vi "Initialise.vi"(8 "error in (no error)":errorcluster, 11 "Actor in":refnum<class "Main View.lvclass">) -> (0 "error out":errorcluster, 3 "Actor out":refnum<class "Main View.lvclass">, 5 "Observers":T1)   [LabVIEW 2015, in "Main View.lvclass"]
uses:
  Main View.lvclass
  Re-use Libraries/Minimal Actor Framework/Messaging/Message/Message.lvclass
  Re-use Libraries/Minimal Actor Framework/Actors/Base Actor/Actor/Update User Event.ctl
  Re-use Libraries/Utility/Utility.lvlib
  Actors/Main Controller/Actor/Main Controller Actor.lvclass
  Re-use Libraries/Minimal Actor Framework/Actors/Base Actor/Actor/Actor.lvclass
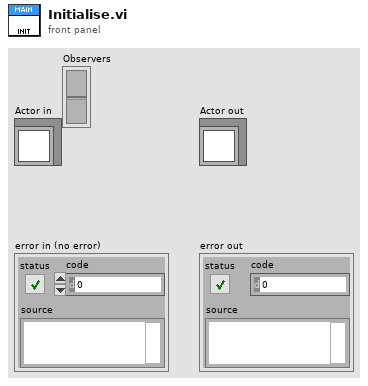
[diagram p1: front panel]
types:
  T1 = cluster{"Actor":refnum<event-registration>, "Main Controller":refnum<event-registration>}
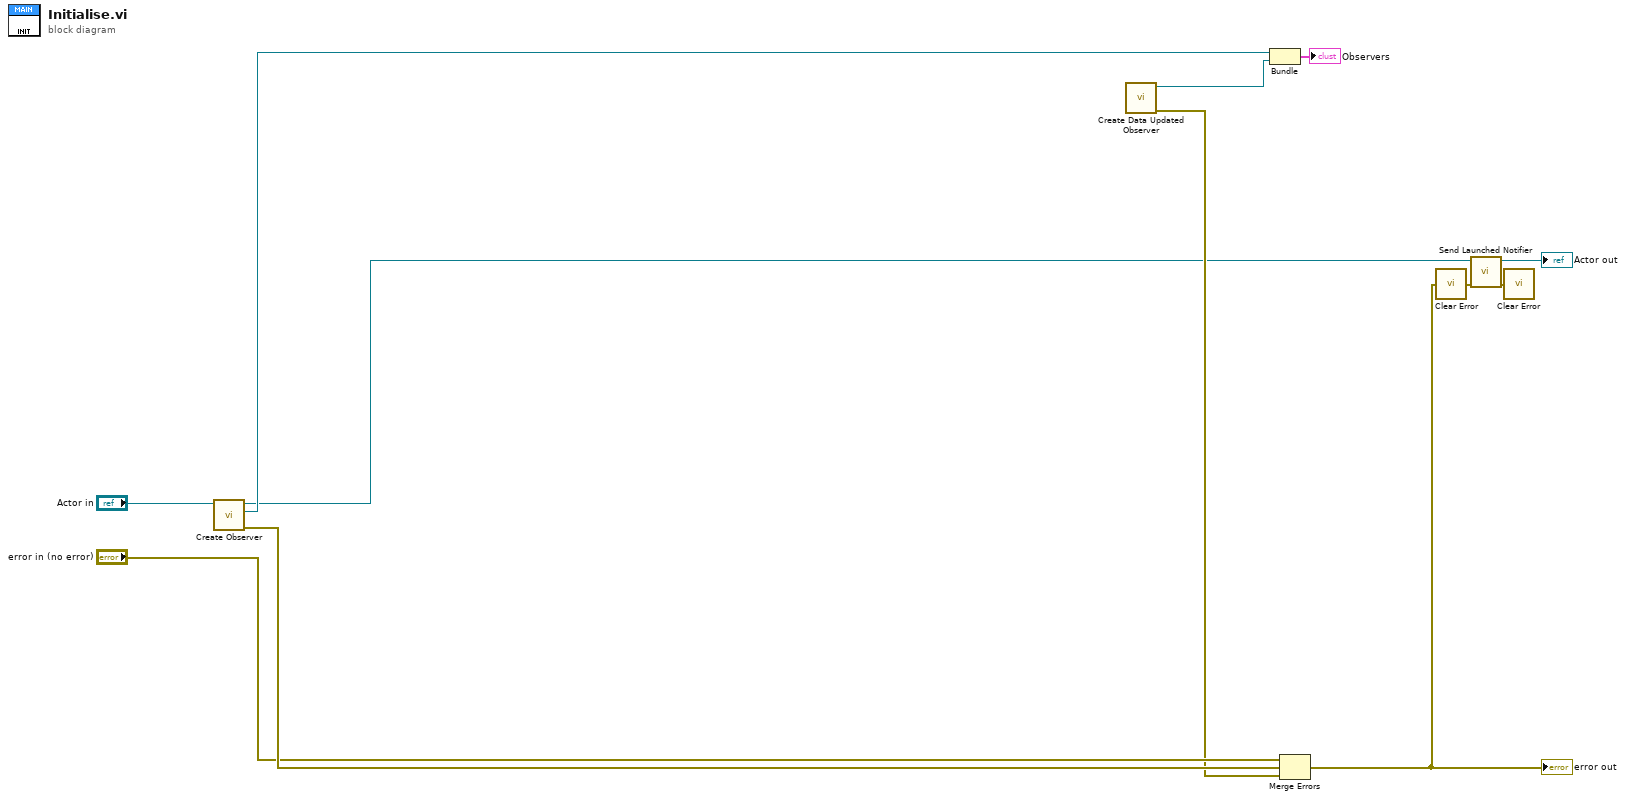
[diagram p0: block diagram]
diagram:
  n1 = call-dynamic "Create Observer.vi"("Actor in"="Actor in") -> ("error out"=w10:errorcluster, "Actor"=w5:refnum<event-registration>, "Actor out"=w1:refnum<class "Main View.lvclass">)  [unwired: 8 in]
  n2 = call "Create Data Updated Observer.vi"() -> ("error out"=w3:errorcluster, "Main Controller"=w4:refnum<event-registration>)  [unwired: 10 in]
  n3 = Bundle("Actor"=w5, "Main Controller"=w4) -> (→"Observers":T1)  [unwired: 1 in]
  n4 = Merge Errors("error in (no error)", w10, w3) -> (w9:errorcluster)
  "error out" <- w9
  n5 = call "Clear Error.vi"("error in (no error)"=w9) -> ("error out"=w8:errorcluster)
  n6 = call-dynamic "Send Launched Notifier.vi"("error in (no error)"=w8, "Actor in"=w1) -> ("error out"=w7:errorcluster, "Actor out"=→"Actor out":refnum<class "Main View.lvclass">)  [unwired: 8 in]
  n7 = call "Clear Error.vi"("error in (no error)"=w7) -> ()  [unwired: 1 out]
